vi "2_1.vi"() -> ()   [LabVIEW 2010]
panel:
  out "I3":dbl
  out "I2":dbl
  out "I1":dbl
  in  "R3":dbl
  in  "R2":dbl
  in  "R1":dbl
  in  "E":dbl
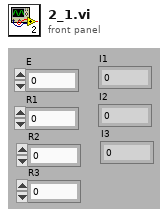
[diagram p1: front panel]
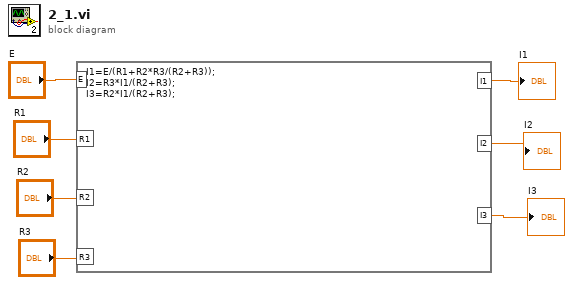
[diagram p0: block diagram]
diagram:
  n1 = formula code="I1=E/(R1+R2*R3/(R2+R3));\nI2=R3*I1/(R2+R3);\nI3=R2*I1/(R2+R3);"("E"="E", "R1"="R1", "R2"="R2", "R3"="R3") -> ("I1"=→"I1":dbl, "I2"=→"I2":dbl, "I3"=→"I3":dbl)
